vi "Plot Editor_Store to Plot Style.vi"(7 "XYGraph in":refnum<vi>, 8 "error in (no error)":errorcluster, 11 "Plot Editor Internal Data":T1) -> (0 "error out":errorcluster, 3 "Plot Editor Internal Data (dup)":T1)   [LabVIEW 2019, in "Plot Editor.lvlib"]
uses:
  Plot Editor.lvlib
  Plot Editor Internal Variables.ctl
  XY Graph/XY Graph Plot Properties.ctl
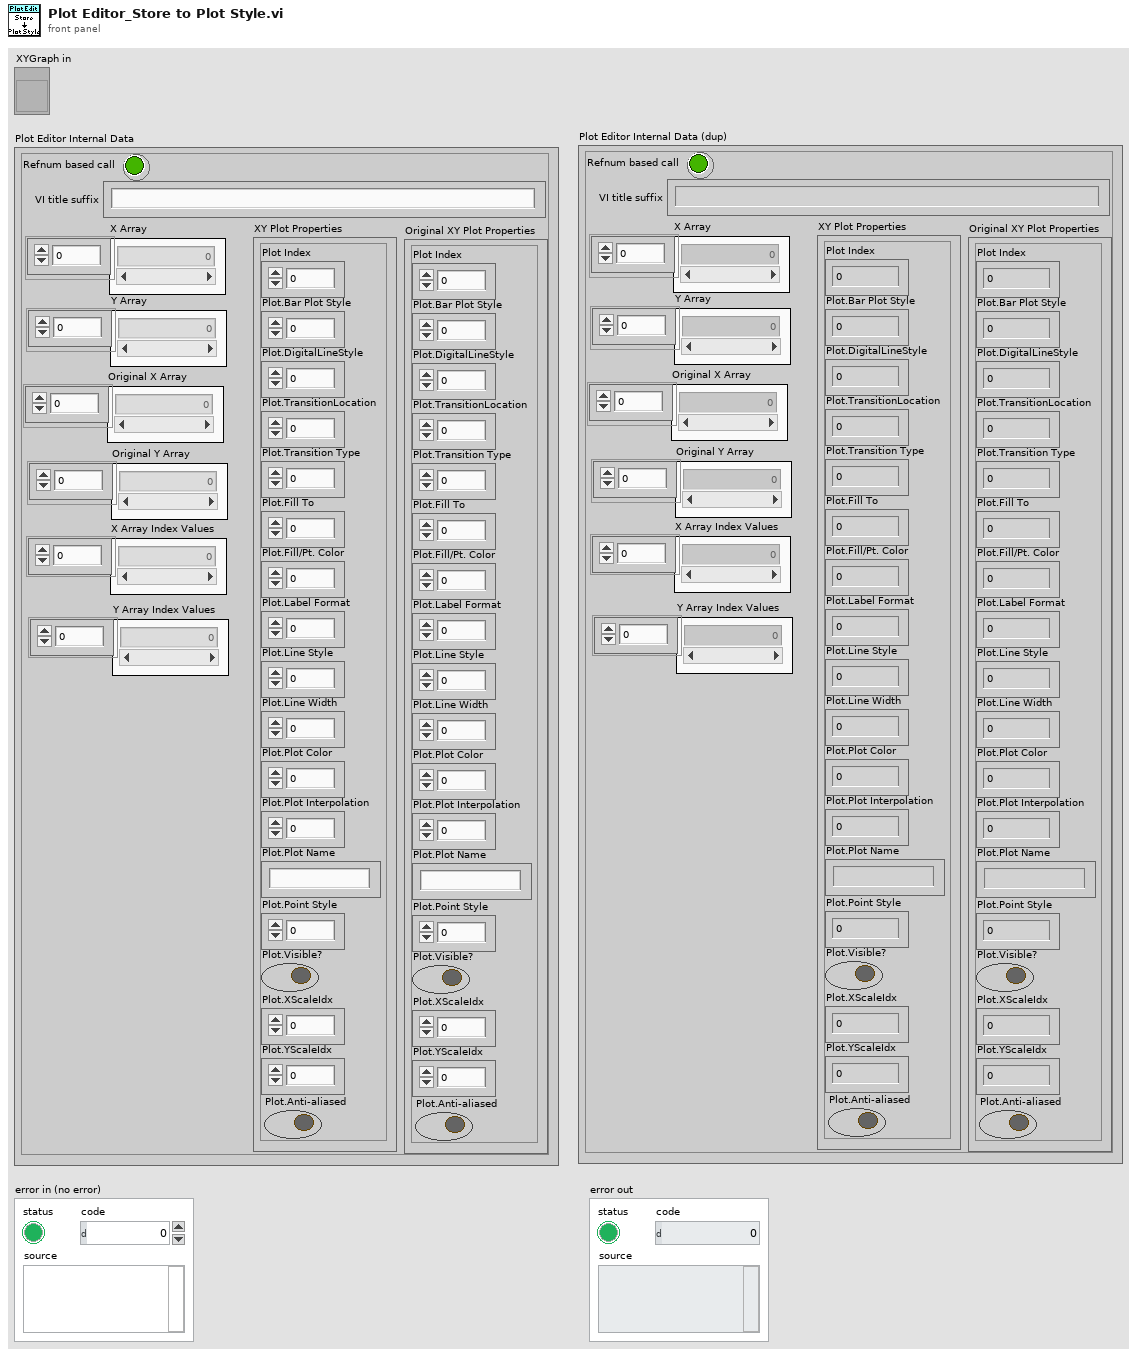
[diagram p1: front panel]
types:
  T1 = typedef "Plot Editor.lvlib/Plot Editor Internal Variables.ctl" = cluster{"X Array":dbl[], "Y Array":dbl[], "XY Plot Properties":T2, "X Array Index Values":u32[], "Y Array Index Values":u32[], "Original XY Plot Properties":T2, "Original X Array":dbl[], "Original Y Array":dbl[], "VI title suffix":string, "Refnum based call":bool}
  T2 = typedef "XY Graph Plot Properties.ctl" = cluster{"Plot Index":i32, "Plot.Bar Plot Style":u8, "Plot.DigitalLineStyle":u8, "Plot.TransitionLocation":u8, "Plot.Transition Type":u8, "Plot.Fill To":i16, "Plot.Fill/Pt. Color":u32, "Plot.Label Format":u8, "Plot.Line Style":u8, "Plot.Line Width":u8, "Plot.Plot Color":u32, "Plot.Plot Interpolation":u8, "Plot.Plot Name":string, "Plot.Point Style":u8, "Plot.Visible?":bool, "Plot.XScaleIdx":u32, "Plot.YScaleIdx":u32, "Plot.Anti-aliased":bool}
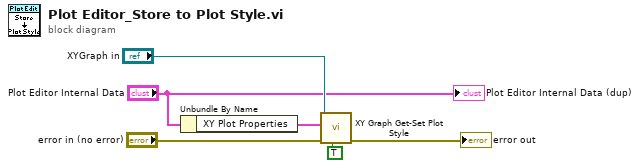
[diagram p0: block diagram]
diagram:
  n1 = Unbundle By Name("Plot Editor Internal Data") -> ("XY Plot Properties"=w4:T2)
  n2 = call "XY Graph Get-Set Plot Style.vi"("Get (F)/Set"=TRUE, "Error In"="error in (no error)", "Plot Style in"=w4, "XYGraph in"="XYGraph in") -> ("Error Out"=→"error out":errorcluster)  [unwired: 4 in, 3 out]
  "Plot Editor Internal Data (dup)" <- "Plot Editor Internal Data"
